vi "log create.vi"(11 "message":string) -> ()   [LabVIEW 2019]
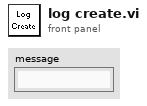
[diagram p1: front panel]
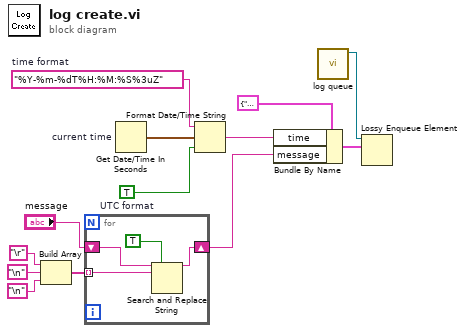
[diagram p0: block diagram]
diagram:
  w10 = TRUE  # UTC format
  w11 = "%Y-%m-%dT%H:%M:%S%3uZ"  # time format
  n1 = Build Array("\r", "\n", "\n") -> (w2:string[])
  n2 = for {
    shift-right: [w17] -> w1
    shift-left: "message" -> [w16]
    tunnel: w2 -> [w15] mode=indexing
    n3 = Search and Replace String(replace all?=TRUE ("replace all? (F)"), input string=w16, search string=w15) -> (result string=w17:string)  [unwired: 5 in, 3 out]
  }
  n4 = Get Date/Time In Seconds "current time"() -> (seconds since 1Jan1904=w12:timestamp)
  n5 = Format Date/Time String(time format string (%c)=w11, seconds (now)=w12, UTC format=w10) -> (date/time string=w8:string)
  n6 = Bundle By Name(cluster=cluster{"time":string, "message":string} {"time"="", "message"=""} ("element"), "time"=w8, "message"=w1) -> (w7:cluster{"time":string, "message":string})
  n7 = call "log queue.vi"() -> ("queue out"=w13:refnum<queue>)  [unwired: 11 in]
  n8 = Lossy Enqueue Element(queue=w13, element=w7) -> ()  [unwired: 1 in, 4 out]
